vi "选择方块.vi"(11 "ID":i8) -> (1 "列":i32, 2 "行":i32, 3 "数组":u32[][](array[colorbox]))   [LabVIEW 2012]
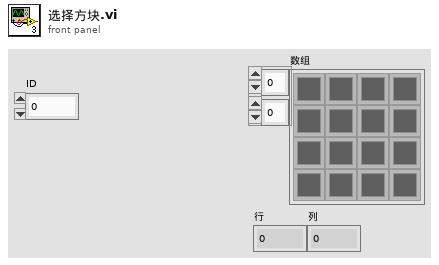
[diagram p1: front panel]
types:
  T1 = cluster{cluster{bool[][], bool[][], bool[][], bool[][], u32}, cluster{bool[][], bool[][], bool[][], bool[][], u32}, cluster{bool[][], bool[][], bool[][], bool[][], u32}, cluster{bool[][], bool[][], u32}, cluster{bool[][], bool[][], u32}, cluster{bool[][], bool[][], u32}, cluster{bool[][], u32}}
  T2 = cluster{bool[][], bool[][], bool[][], bool[][], u32}
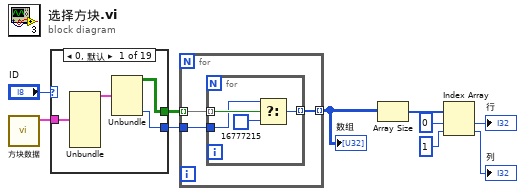
[diagram p0: block diagram]
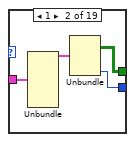
[diagram p2: hidden frame]
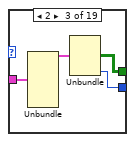
[diagram p3: hidden frame]
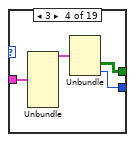
[diagram p4: hidden frame]
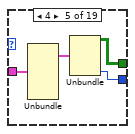
[diagram p5: hidden frame]
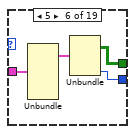
[diagram p6: hidden frame]
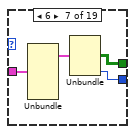
[diagram p7: hidden frame]
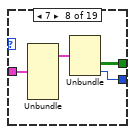
[diagram p8: hidden frame]
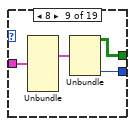
[diagram p9: hidden frame]
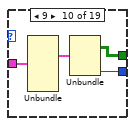
[diagram p10: hidden frame]
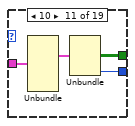
[diagram p11: hidden frame]
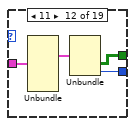
[diagram p12: hidden frame]
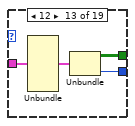
[diagram p13: hidden frame]
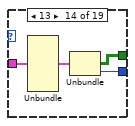
[diagram p14: hidden frame]
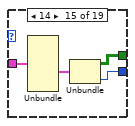
[diagram p15: hidden frame]
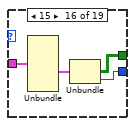
[diagram p16: hidden frame]
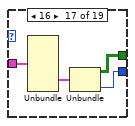
[diagram p17: hidden frame]
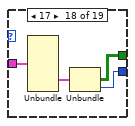
[diagram p18: hidden frame]
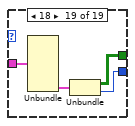
[diagram p19: hidden frame]
diagram:
  n1 = call "方块数据.vi"() -> ("输出簇"=w9:T1)  [unwired: 11 in]
  n2 = case shown="0, 默认" "ID" {
    tunnel: [w12 w16 w20 w24 w28 w32 w36 w40 w44 w48 w52 w56 w60 w64 w68 w72 w76 w80 w84] -> w7
    tunnel: [w11 w15 w19 w23 w27 w31 w35 w39 w43 w47 w51 w55 w59 w63 w67 w71 w75 w79 w83] -> w8
    tunnel: w9 -> [w14 w18 w22 w26 w30 w34 w38 w42 w46 w50 w54 w58 w62 w66 w70 w74 w78 w82 w86]
    frame 0, Default {
      n3 = Unbundle(w14) -> (w13:T2)  [unwired: 6 out]
      n4 = Unbundle(w13) -> (w12:bool[][], w11:u32)  [unwired: 3 out]
    }
    frame 1 {
      n5 = Unbundle(w18) -> (w17:T2)  [unwired: 6 out]
      n6 = Unbundle(w17) -> (w16:bool[][], w15:u32)  [unwired: 3 out]
    }
    frame 2 {
      n7 = Unbundle(w22) -> (w21:T2)  [unwired: 6 out]
      n8 = Unbundle(w21) -> (w20:bool[][], w19:u32)  [unwired: 3 out]
    }
    frame 3 {
      n9 = Unbundle(w26) -> (w25:T2)  [unwired: 6 out]
      n10 = Unbundle(w25) -> (w24:bool[][], w23:u32)  [unwired: 3 out]
    }
    frame 4 {
      n11 = Unbundle(w30) -> (w29:T2)  [unwired: 6 out]
      n12 = Unbundle(w29) -> (w28:bool[][], w27:u32)  [unwired: 3 out]
    }
    frame 5 {
      n13 = Unbundle(w34) -> (w33:T2)  [unwired: 6 out]
      n14 = Unbundle(w33) -> (w32:bool[][], w31:u32)  [unwired: 3 out]
    }
    frame 6 {
      n15 = Unbundle(w38) -> (w37:T2)  [unwired: 6 out]
      n16 = Unbundle(w37) -> (w36:bool[][], w35:u32)  [unwired: 3 out]
    }
    frame 7 {
      n17 = Unbundle(w42) -> (w41:T2)  [unwired: 6 out]
      n18 = Unbundle(w41) -> (w40:bool[][], w39:u32)  [unwired: 3 out]
    }
    frame 8 {
      n19 = Unbundle(w46) -> (w45:T2)  [unwired: 6 out]
      n20 = Unbundle(w45) -> (w44:bool[][], w43:u32)  [unwired: 3 out]
    }
    frame 9 {
      n21 = Unbundle(w50) -> (w49:T2)  [unwired: 6 out]
      n22 = Unbundle(w49) -> (w48:bool[][], w47:u32)  [unwired: 3 out]
    }
    frame 10 {
      n23 = Unbundle(w54) -> (w53:T2)  [unwired: 6 out]
      n24 = Unbundle(w53) -> (w52:bool[][], w51:u32)  [unwired: 3 out]
    }
    frame 11 {
      n25 = Unbundle(w58) -> (w57:T2)  [unwired: 6 out]
      n26 = Unbundle(w57) -> (w56:bool[][], w55:u32)  [unwired: 3 out]
    }
    frame 12 {
      n27 = Unbundle(w62) -> (w61:cluster{bool[][], bool[][], u32})  [unwired: 6 out]
      n28 = Unbundle(w61) -> (w60:bool[][], w59:u32)  [unwired: 1 out]
    }
    frame 13 {
      n29 = Unbundle(w66) -> (w65:cluster{bool[][], bool[][], u32})  [unwired: 6 out]
      n30 = Unbundle(w65) -> (w64:bool[][], w63:u32)  [unwired: 1 out]
    }
    frame 14 {
      n31 = Unbundle(w70) -> (w69:cluster{bool[][], bool[][], u32})  [unwired: 6 out]
      n32 = Unbundle(w69) -> (w68:bool[][], w67:u32)  [unwired: 1 out]
    }
    frame 15 {
      n33 = Unbundle(w74) -> (w73:cluster{bool[][], bool[][], u32})  [unwired: 6 out]
      n34 = Unbundle(w73) -> (w72:bool[][], w71:u32)  [unwired: 1 out]
    }
    frame 16 {
      n35 = Unbundle(w78) -> (w77:cluster{bool[][], bool[][], u32})  [unwired: 6 out]
      n36 = Unbundle(w77) -> (w76:bool[][], w75:u32)  [unwired: 1 out]
    }
    frame 17 {
      n37 = Unbundle(w82) -> (w81:cluster{bool[][], bool[][], u32})  [unwired: 6 out]
      n38 = Unbundle(w81) -> (w80:bool[][], w79:u32)  [unwired: 1 out]
    }
    frame 18 {
      n39 = Unbundle(w86) -> (w85:cluster{bool[][], u32})  [unwired: 6 out]
      n40 = Unbundle(w85) -> (w84:bool[][], w83:u32)
    }
  }
  n41 = for {
    tunnel: w7 -> [w89] mode=indexing
    tunnel: w8 -> [w88]
    tunnel: [w87] -> w6 mode=indexing
    n42 = for {
      tunnel: w89 -> [w93] mode=indexing
      tunnel: w88 -> [w92]
      tunnel: [w90] -> w87 mode=indexing
      n43 = Select(t=w92, s=w93, f=u32 16777215) -> (s? t:f=w90:u32)
    }
  }
  "数组" <- w6
  n44 = Array Size(array=w6) -> (size(s)=w5:i32[])
  n45 = Index Array(array=w5, index #1=0 ("索引"), index #2=1 ("索引")) -> (element #1=→"行":i32, element #2=→"列":i32)
